vi "Network Sync.vi"(8 "error in (no error)":errorcluster, 10 "Timeout (5000 ms)":dbl=5000.0, 11 "MatlabExperiment in":refnum<class "MatlabExperiment.lvclass">) -> (0 "error out":errorcluster, 3 "MatlabExperiment out":refnum<class "MatlabExperiment.lvclass">)   [LabVIEW 2014, in "AcquisitionCoreObjects.lvlib" / "MatlabExperiment.lvclass"]
uses:
  MatlabExperiment.lvclass
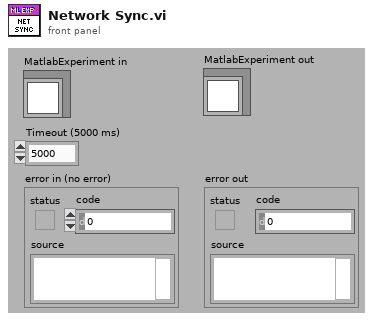
[diagram p1: front panel]
types:
  T1 = enum16{"Get Time", "Get Elapsed Time", "Reset Elapsed Time"}
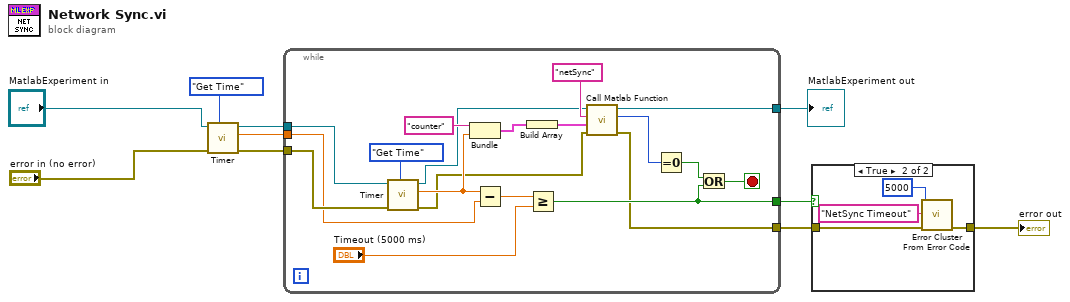
[diagram p0: block diagram]
diagram:
  n1 = call-dynamic "Timer.vi"("Method"=T1."Get Time", "error in (no error)"="error in (no error)", "BehaviorData in"="MatlabExperiment in") -> ("error out"=w9:errorcluster, "Time"=w7:dbl, "BehaviorData out"=w8:refnum<class "MatlabExperiment.lvclass">)  [unwired: 5 in, 1 out]
  n2 = while {
    tunnel: w9 -> [w26]
    tunnel: w8 -> [w27]
    tunnel: w7 -> [w25]
    tunnel: [w19] -> w6
    tunnel: [w13] -> w4
    tunnel: [w12] -> w3
    stop <- w22 stop-if-true
    n3 = call-dynamic "Timer.vi"("Method"=T1."Get Time", "error in (no error)"=w26, "BehaviorData in"=w27) -> ("error out"=w14:errorcluster, "Time"=w16:dbl, "BehaviorData out"=w11:refnum<class "MatlabExperiment.lvclass">)  [unwired: 5 in, 1 out]
    n4 = Bundle("counter", "Time"=w16) -> (w18:cluster{string, "Time":dbl})  [unwired: 1 out]
    n5 = Subtract(x=w16, y=w25) -> (x-y=w24:dbl)
    n6 = Build Array(w18) -> (w15:cluster{string, "Time":dbl}[])
    n7 = Greater Or Equal?(x=w24, y="Timeout (5000 ms)") -> (x >= y?=w13:bool)
    n8 = call-dynamic "Call Matlab Function.vi"("error in (no error)"=w14, "Matlab Param Array"=w15, "Function name"="netSync", "TrialBasedExperiment in"=w11) -> ("error out"=w12:errorcluster, "Return value I32"=w21:i32, "TrialBasedExperiment out"=w19:refnum<class "MatlabExperiment.lvclass">)  [unwired: 4 in, 1 out]
    n9 = Equal To 0?(x=w21) -> (x = 0?=w20:bool)
    n10 = Or(x=w20, y=w13) -> (x .or. y?=w22:bool)
  }
  "MatlabExperiment out" <- w6
  n11 = case shown="True" w4 {
    tunnel: [w30 w32] -> w5
    tunnel: w3 -> [w30 w31]
    frame False {
    }
    frame True {
      n12 = call <vilib>:"Error Cluster From Error Code.vi"("error in (no error)"=w31, "error message (\"\")"="NetSync Timeout" ("error message (\"\")"), "error code (0)"=5000) -> ("error out"=w32:errorcluster)  [unwired: 6 in]
    }
  }
  "error out" <- w5
